vi "S2C_Access_Initialize.vi"(8 "Error In":errorcluster, 11 "DSN Path":path) -> (0 "Error Out":errorcluster)   [LabVIEW 2015]
uses:
  S2C_Access_Globals.vi
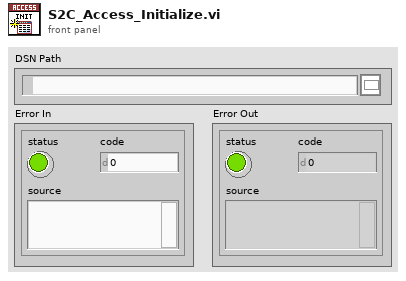
[diagram p1: front panel]
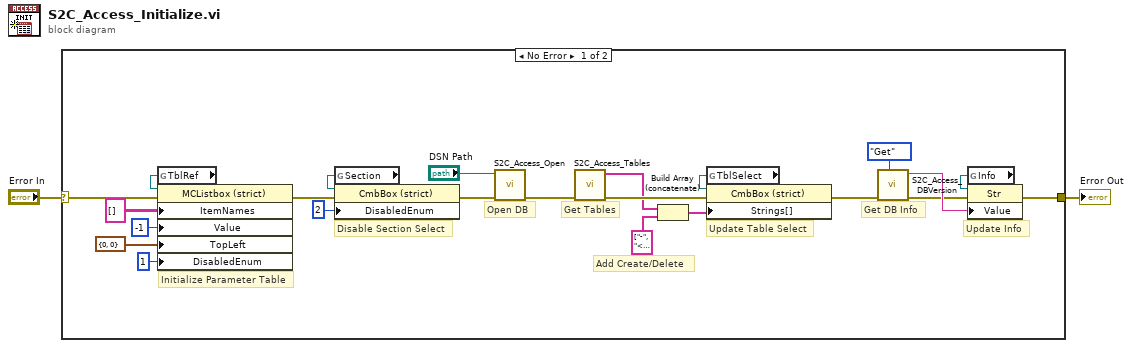
[diagram p0: block diagram]
diagram:
  n1 = case shown="No Error" "Error In" {
    selector: "Error In" -> [w25 w26]
    tunnel: [w10 w26] -> w1
    frame No Error {
      # "Add Create/Delete"
      # "Update Info"
      # "Get DB Info"
      # "Update Table Select"
      # "Get Tables"
      # "Open DB"
      # "Disable Section Select"
      # "Initialize Parameter Table"
      n2 = global read "S2C_Access_Globals.vi" "TblRef"() -> (w24:refnum<vi>)
      n3 = property class="MCListbox (strict)"(reference=w24, error in=w25, "ItemNames"=string[][] [] ("Item Names"), "Value"=-1 ("ParamTbl"), "TopLeft"=cluster{"Row":u32, "Column":u32} {"Row"=0, "Column"=0} ("Top Left Visible Cell"), "DisabledEnum"=1) -> (error out=w18:errorcluster)  [unwired: 1 out]
      n4 = global read "S2C_Access_Globals.vi" "Section"() -> (w19:refnum<vi>)
      n5 = property class="CmbBox (strict)"(reference=w19, error in=w18, "DisabledEnum"=2) -> (error out=w7:errorcluster)  [unwired: 1 out]
      n6 = call "S2C_Access_Open.vi"("Error In"=w7, "DSN_Path"="DSN Path") -> ("Error Out"=w16:errorcluster)  [unwired: 8 in, 1 out]
      n7 = call "S2C_Access_Tables.vi"("Error In"=w16) -> ("Error Out"=w14:errorcluster, "Tables"=w6:string[])  [unwired: 9 in]
      n8 = Build Array (concatenate)(w6, string[] ["-", "<Create Table>", "<Delete Table>"]) -> (w5:string[])
      n9 = global read "S2C_Access_Globals.vi" "TblSelect"() -> (w15:refnum<vi>)
      n10 = property class="CmbBox (strict)"(reference=w15, error in=w14, "Strings[]"=w5) -> (error out=w12:errorcluster)  [unwired: 1 out]
      n11 = call "S2C_Access_DBVersion.vi"("Action"=enum16{"Get", "Set"}."Get", "Error In"=w12) -> ("Error Out"=w8:errorcluster, "Data Out"=w9:string)  [unwired: 8 in]
      n12 = global read "S2C_Access_Globals.vi" "Info"() -> (w11:refnum<vi>)
      n13 = property class="Str"(reference=w11, error in=w8, "Value"=w9) -> (error out=w10:errorcluster)  [unwired: 1 out]
    }
    frame Error {
    }
  }
  "Error Out" <- w1
